vi "RemoveInvalidValues.vi"(11 "In":dbl) -> (3 "Out":dbl)   [LabVIEW 2024]
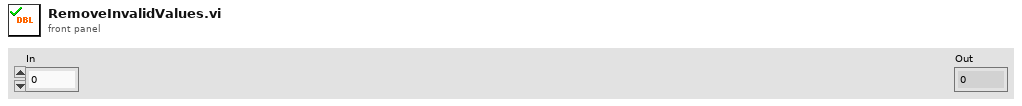
[diagram p1: front panel]
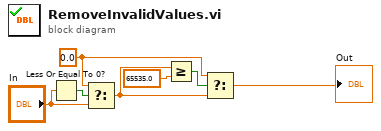
[diagram p0: block diagram]
diagram:
  w4 = 0.0 ("t")
  n1 = Less Or Equal To 0?(x="In") -> (x <= 0?=w7:bool)
  n2 = Select(t=w4, s=w7, f="In") -> (s? t:f=w3:dbl)
  n3 = Greater Or Equal?(x=w3, y=65535.0) -> (x >= y?=w5:bool)
  n4 = Select(t=w4, s=w5, f=w3) -> (s? t:f=→"Out":dbl)
